vi "InfoAndSetupPage.vi"() -> ()   [LabVIEW 2026]
panel:
  out "Machine Status":T1
  out "Overscan Steps (%)":string
  in  "Use Calculated Diameter":bool
  in  "Calculate Scan":bool
  in  "Scan Settings":T2
  in  "Cluster 2":T3
  in  "Scan information":T4
  in  "Transducer Information":string[][](table)
  # "Scan Settings"
  # "Scan Information"
  # "Machine Status"
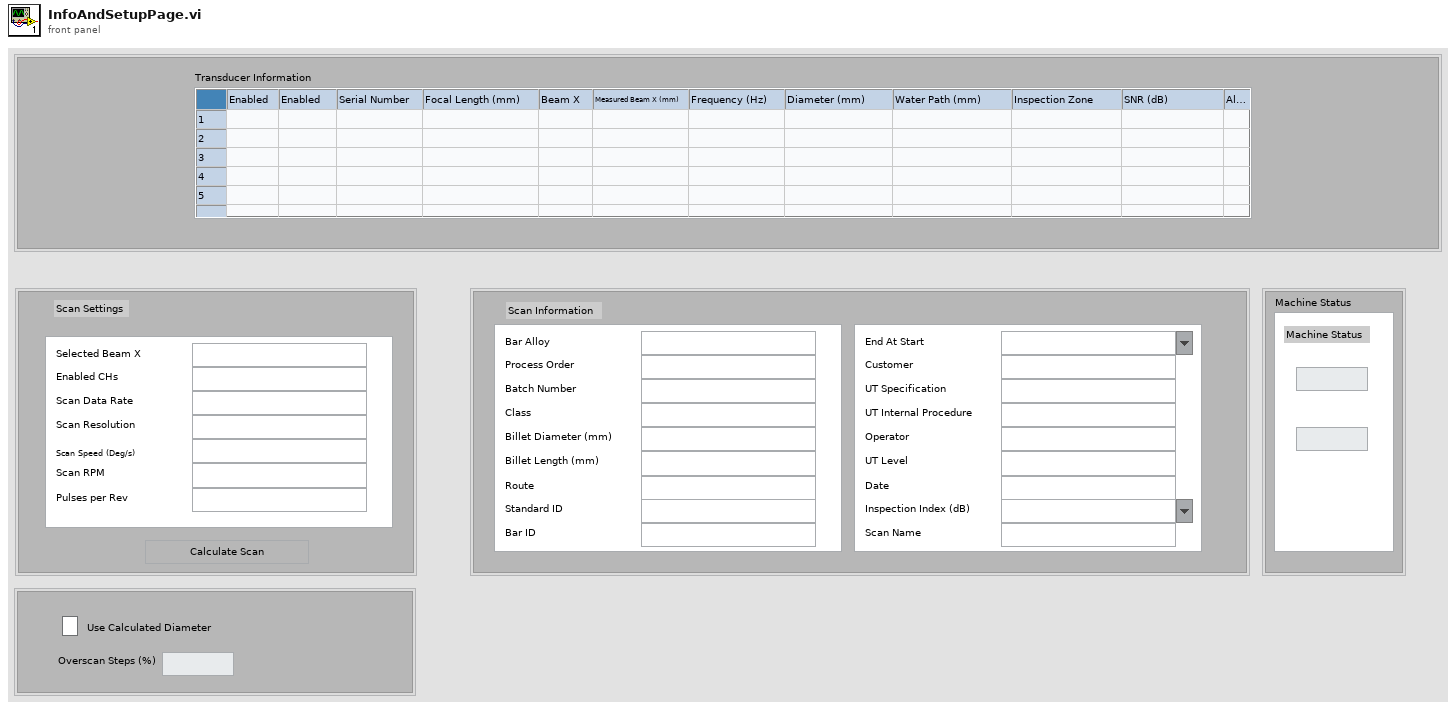
[diagram p1: front panel]
types:
  T1 = cluster{"MachineState1\nMachineState1":string, "Machine State 2":string}
  T2 = cluster{"Selected Beam X":string, "Enabled CHs":string, "Scan Data Rate":string, "Scan Resolution":string, "\nScan Speed (Deg/s)":string, "Scan RPM":string, "Pulses per Rev":string}
  T3 = cluster{"End At Start":string, "Customer":string, "UT Specification":string, "UT Internal Procedure":string, "Operator":string, "UT Level":string, "Date":string, "Inspection Index (dB)":string, "Scan Name":string}
  T4 = cluster{"Bar Alloy\n":string, "Process Order":string, "Batch Number":string, "Class":string, "Billet Diameter (mm)":string, "Billet Length (mm)":string, "Route":string, "Standard ID":string, "Bar ID":string}
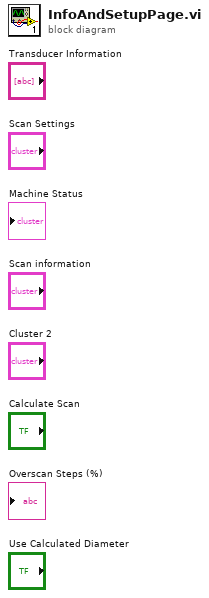
[diagram p0: block diagram]
diagram:
